vi "Launch Datalogger.vi"(8 "error in":errorcluster, 11 "Instruments in":refnum<class "Instruments.lvclass">) -> (0 "error out":errorcluster, 3 "Instruments out":refnum<class "Instruments.lvclass">)   [LabVIEW 2023, in "Instruments.lvlib" / "Instruments.lvclass"]
uses:
  Library/Instruments.lvclass
  C:/Users/Public/Documents/Development/builds/Engine/Engine.lvlibp/Project/Engine.lvclass
  C:/Users/Public/Documents/Development/builds/Engine/Actor Framework.lvlibp/1abvi3w/vi.lib/ActorFramework/Actor/Actor.lvclass
  builds/Engine/Engine.lvlibp/Accessors/Read Report Queue.vi
  builds/Engine/Actor Framework.lvlibp/1abvi3w/vi.lib/ActorFramework/Actor/Read Actor Label.vi
  builds/Tools/QDMH.lvlibp/Private/Enqueue Bundled Element.vi
  builds/Engine/Engine.lvlibp/Accessors/Write Report Queue.vi
  builds/Tools/QDMH.lvlibp/QDMH.lvclass
  builds/Engine/Engine.lvlibp/Project/Engine.lvclass
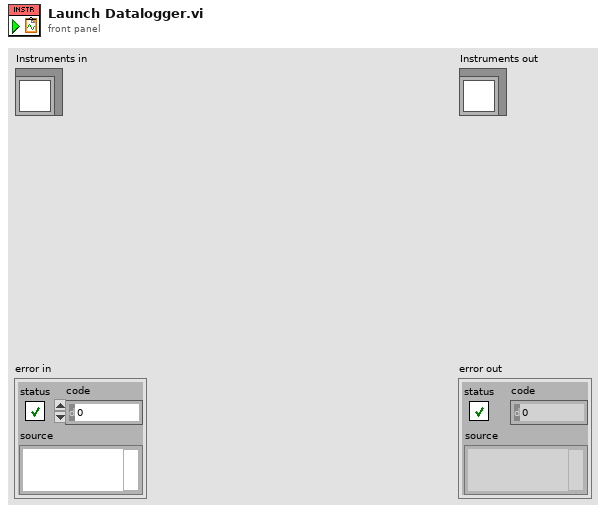
[diagram p1: front panel]
types:
  T1 = cluster{"Accessors:Actor Label":string, string[], variant[]}
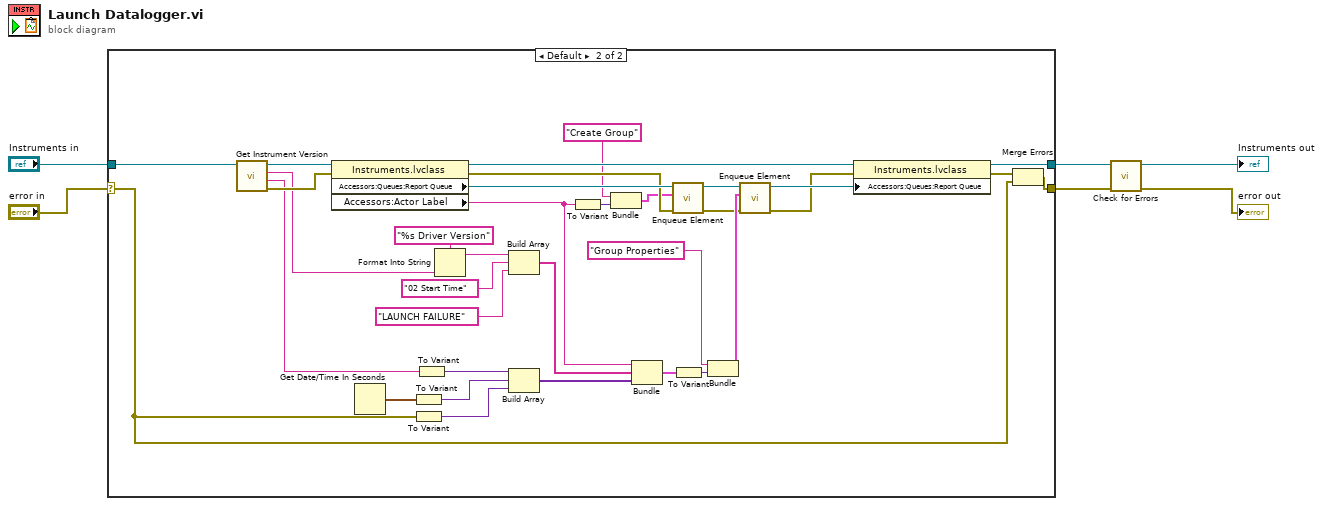
[diagram p0: block diagram]
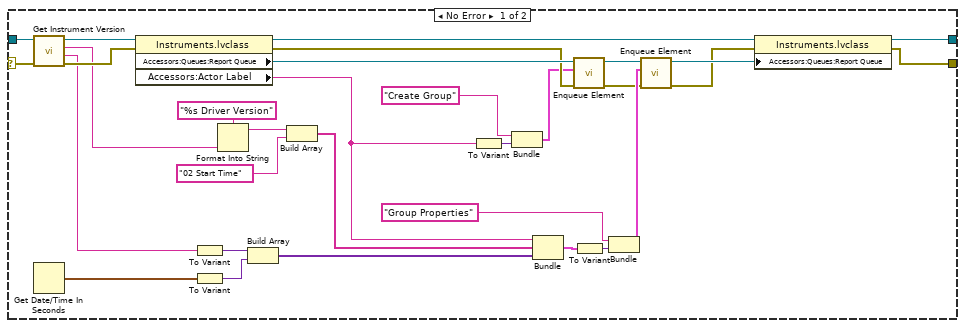
[diagram p2: hidden frame]
diagram:
  n1 = case shown="Default" "error in" {
    selector: "error in" -> [w19 w39]
    tunnel: [w37 w71] -> w4
    tunnel: [w36 w41] -> w3
    tunnel: "Instruments in" -> [w18 w54]
    frame No Error {
      n2 = call "Get Instrument Version.vi"("error in"=w19, "Instruments in"=w18) -> ("error out"=w26:errorcluster, "Version"=w21:string, "Driver"=w20:string, "Instruments out"=w27:refnum<class "Instruments.lvclass">)  [unwired: 6 in]
      n3 = Get Date/Time In Seconds() -> (seconds since 1Jan1904=w9:timestamp)
      n4 = property class="Instruments.lvclass"(reference=w27, error in=w26) -> (reference out=w25:refnum<class "Instruments.lvclass">, error out=w12:errorcluster, "Accessors:Queues:Report Queue"=w17:refnum<class "QDMH.lvclass">, "Accessors:Actor Label"=w14:string)
      n5 = To Variant(anything=w21) -> (Variant=w31:variant)
      n6 = To Variant(anything=w9) -> (Variant=w8:variant)
      n7 = Format Into String(format string="%s Driver Version", w20) -> (resulting string=w33:string)  [unwired: 2 in, 1 out]
      n8 = Build Array(w31, w8) -> (w30:variant[])
      n9 = Build Array(w33, "02 Start Time" ("element")) -> (w32:string[])
      n10 = To Variant(anything=w14) -> (Variant=w13:variant)
      n11 = Bundle("Create Group", "Variant"=w13) -> (w11:cluster{string, "Variant":variant})  [unwired: 1 in]
      n12 = Bundle("Accessors:Actor Label"=w14, w32, w30) -> (w29:T1)  [unwired: 1 in]
      n13 = call-poly "Enqueue Element.vi"("error in"=w12, "element"=w11, "QDMH in"=w17) -> ("error out"=w15:errorcluster, "QDMH out"=w16:refnum<class "QDMH.lvclass">)  [unwired: 7 in]
      n14 = To Variant(anything=w29) -> (Variant=w24:variant)
      n15 = Bundle("Group Properties", "Variant"=w24) -> (w22:cluster{string, "Variant":variant})  [unwired: 1 in]
      n16 = call-poly "Enqueue Element.vi"("error in"=w15, "element"=w22, "QDMH in"=w16) -> ("error out"=w28:errorcluster, "QDMH out"=w35:refnum<class "QDMH.lvclass">)  [unwired: 7 in]
      n17 = property class="Instruments.lvclass"(reference=w25, error in=w28, "Accessors:Queues:Report Queue"=w35) -> (reference out=w37:refnum<class "Instruments.lvclass">, error out=w36:errorcluster)
    }
    frame Default {
      n18 = call "Get Instrument Version.vi"("Instruments in"=w54) -> ("error out"=w61:errorcluster, "Version"=w56:string, "Driver"=w55:string, "Instruments out"=w62:refnum<class "Instruments.lvclass">)  [unwired: 7 in]
      n19 = property class="Instruments.lvclass"(reference=w62, error in=w61) -> (reference out=w60:refnum<class "Instruments.lvclass">, error out=w48:errorcluster, "Accessors:Queues:Report Queue"=w53:refnum<class "QDMH.lvclass">, "Accessors:Actor Label"=w50:string)
      n20 = Get Date/Time In Seconds() -> (seconds since 1Jan1904=w45:timestamp)
      n21 = To Variant(anything=w45) -> (Variant=w44:variant)
      n22 = To Variant(anything=w39) -> (Variant=w38:variant)
      n23 = To Variant(anything=w56) -> (Variant=w66:variant)
      n24 = Format Into String(format string="%s Driver Version", w55) -> (resulting string=w68:string)  [unwired: 2 in, 1 out]
      n25 = Build Array(w68, "02 Start Time" ("element"), "LAUNCH FAILURE" ("element")) -> (w67:string[])
      n26 = Build Array(w66, w44, w38) -> (w65:variant[])
      n27 = To Variant(anything=w50) -> (Variant=w49:variant)
      n28 = Bundle("Create Group", "Variant"=w49) -> (w47:cluster{string, "Variant":variant})  [unwired: 1 in]
      n29 = Bundle("Accessors:Actor Label"=w50, w67, w65) -> (w64:T1)  [unwired: 1 in]
      n30 = call-poly "Enqueue Element.vi"("error in"=w48, "element"=w47, "QDMH in"=w53) -> ("error out"=w51:errorcluster, "QDMH out"=w52:refnum<class "QDMH.lvclass">)  [unwired: 7 in]
      n31 = To Variant(anything=w64) -> (Variant=w59:variant)
      n32 = Bundle("Group Properties", "Variant"=w59) -> (w57:cluster{string, "Variant":variant})  [unwired: 1 in]
      n33 = call-poly "Enqueue Element.vi"("error in"=w51, "element"=w57, "QDMH in"=w52) -> ("error out"=w63:errorcluster, "QDMH out"=w70:refnum<class "QDMH.lvclass">)  [unwired: 7 in]
      n34 = property class="Instruments.lvclass"(reference=w60, error in=w63, "Accessors:Queues:Report Queue"=w70) -> (reference out=w71:refnum<class "Instruments.lvclass">, error out=w42:errorcluster)
      n35 = Merge Errors(w42, w39) -> (w41:errorcluster)
    }
  }
  n36 = call "Check for Errors.vi"("error in"=w3, "Engine in"=w4) -> ("error out"=→"error out":errorcluster, "Engine out"=→"Instruments out":refnum<class "Instruments.lvclass">)  [unwired: 8 in]
